vi "Get events.vi"(0 "Display State In":T1, 9 "Container State":T4, 11 "error in (no error)":errorcluster) -> (4 "Display State Out":T1, 6 "Events":cluster{"Type changed":refnum<user-event>}, 15 "error out":errorcluster)   [LabVIEW 2015, in "PXISlotGP.xctl"]
uses:
  PXISlotGP.xctl
  <vilib>/_xctls/Container State.ctl
  State.ctl
  PXISlot XControl/Connector Type.ctl
  AOAIRefs.ctl
  <vilib>/_xctls/XControlSupport.lvlib
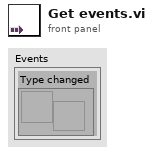
[diagram p1: front panel]
types:
  T1 = typedef "PXISlotGP.xctl/State.ctl" = cluster{"Connector Type":T2, "Hide unused":bool, "Trigger Visible":bool, "TabRef":refnum<vi>, "ConnRefs":refnum<vi>[], "PaneRef":refnum<vi>, "AOAIRefs":T3[], "TriggerRefs":refnum<vi>[], "check data":bool, "Name":string, "Events":cluster{"Type changed":refnum<user-event>}}
  T2 = typedef "Connector Type.ctl" = enum16{"None", "PXI-4461", "BNC-2110", "BNC-2090", "PXIe-4463", "PXIe-4464"}
  T3 = typedef "AOAIRefs.ctl" = cluster{"AORefs":refnum<vi>[], "AIRefs":refnum<vi>[]}
  T4 = typedef "XControlSupport.lvlib/Container State.ctl" = cluster{"Indicator?":bool, "Run Mode?":bool, " Refnum":refnum<vi>}
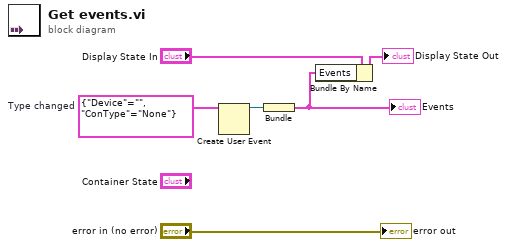
[diagram p0: block diagram]
diagram:
  w3 = cluster{"Device":string, "ConType":T2} {"Device"="", "ConType"=enum."None"}  # Type changed
  n1 = Create User Event(user event datatype=w3) -> (user event=w4:refnum<user-event>)  [unwired: 1 in, 1 out]
  n2 = Bundle("Type changed"=w4) -> (w1:cluster{"Type changed":refnum<user-event>})  [unwired: 1 in]
  "Events" <- w1
  n3 = Bundle By Name(cluster="Display State In", "Events"=w1) -> (→"Display State Out":T1)
  "error out" <- "error in (no error)"
